vi "Spawn.vi"(9 "UID":string, 10 "Actor":refnum<class "Actor.lvclass">, 11 "Base Actor in":refnum<class "Base Actor.lvclass">) -> (0 "Error out":errorcluster, 3 "Base Actor out":refnum<class "Base Actor.lvclass">)   [LabVIEW 2025, in "jettl.lvlib" / "Actor.lvlib" / "Base Actor.lvclass"]
uses:
  Base Actor.lvclass
  Base Actor.lvclass/Base Actor.ctl
  Actor.vi
  Attributes/Attributes/Attributes.lvclass
  Spawn.ctl
  Actor.lvlib
  Actor/Actor.lvclass
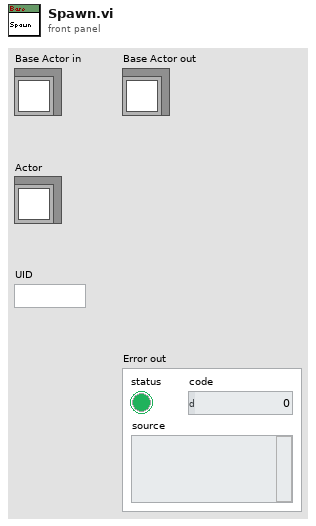
[diagram p1: front panel]
types:
  T1 = typedef "jettl.lvlib/Actor.lvlib/Spawn.ctl" = cluster{"UID":string, "Parent Attributes":refnum<class "Attributes.lvclass">, "Queue of Self Attributes":refnum<queue>, "Queue of Error":refnum<queue>}
  T2 = typedef "jettl.lvlib/Actor.lvlib/Base Actor.lvclass/Child Attributes Map.ctl" = map{string, refnum<class "Attributes.lvclass">}
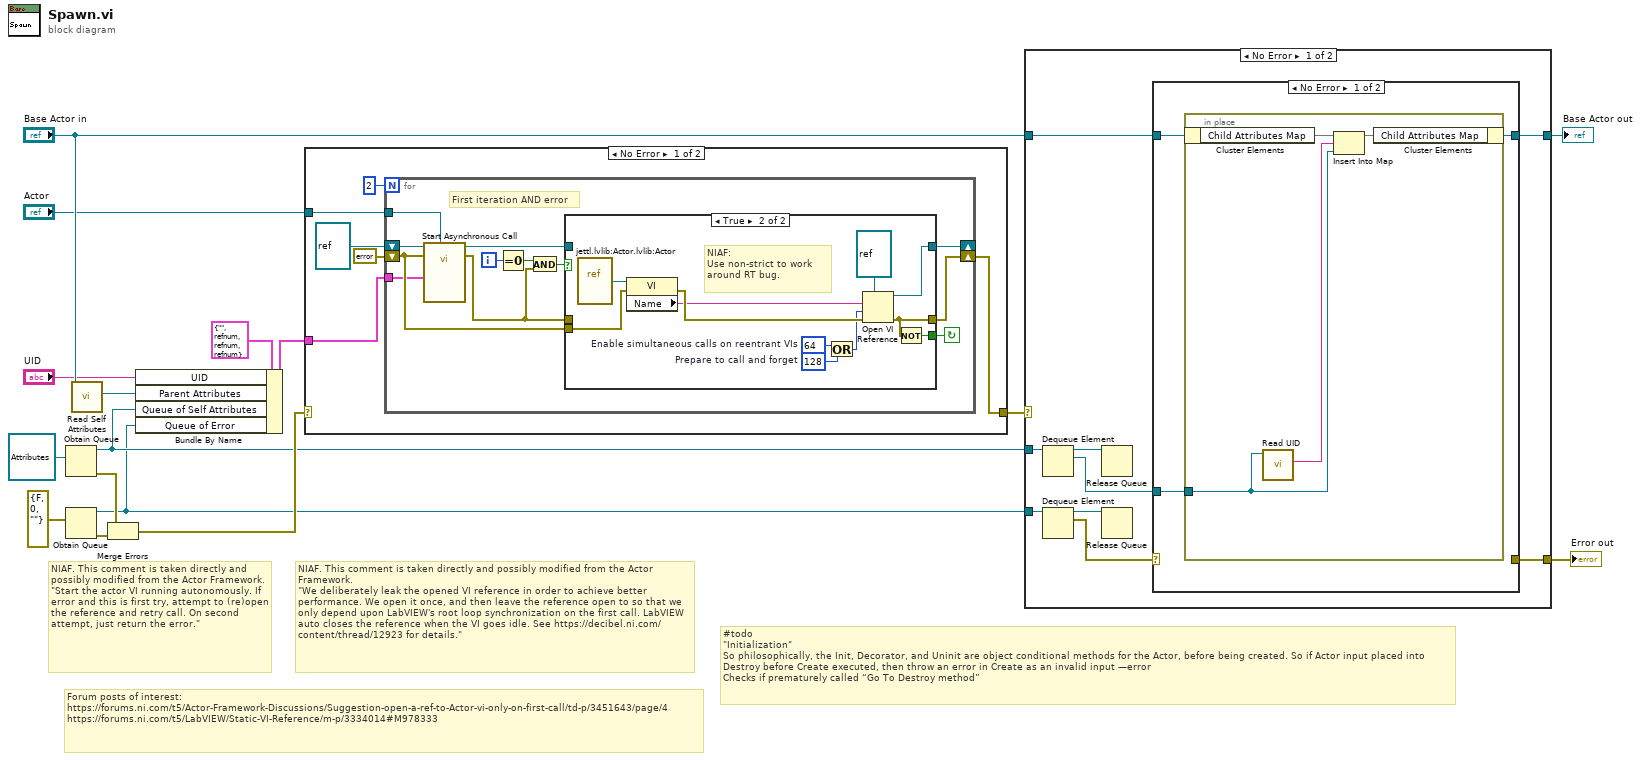
[diagram p0: block diagram]
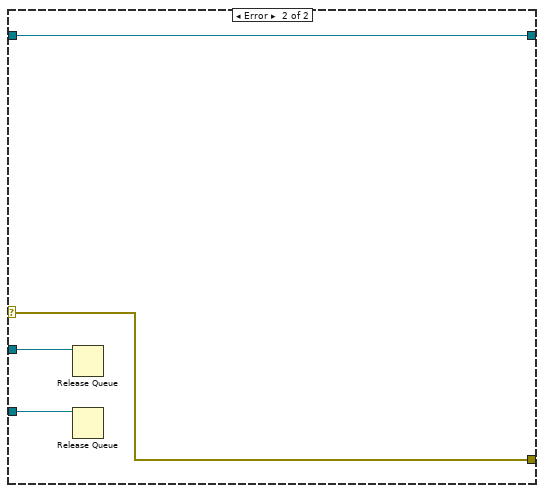
[diagram p3: hidden frame]
diagram:
  # "Forum posts of interest:\nhttps://forums.ni.com/t5/Actor-Framework-Discussions/Suggestion-open-a-ref-to-Actor-vi-only-on-first-call/td-p/3451643/page/4\nhttps://forums.ni.com/t5/LabVIEW/Static-VI-Reference/m-p/3334014#M978333"
  # "NIAF. This comment is taken directly and possibly modified from the Actor Framework.\n\"We deliberately leak the opened VI reference in order to achieve better performance. We open it once, and then leave the reference open to so that we only depend upon LabVIEW's root loop synchronization on the first call. LabVIEW auto closes the reference when the VI goes idle. See https://decibel.ni.com/content/thread/12923 for details.\""
  # "NIAF. This comment is taken directly and possibly modified from the Actor Framework.\n\"Start the actor VI running autonomously. If error and this is first try, attempt to (re)open the reference and retry call. On second attempt, just return the error.\""
  # "#todo\n\"Initialization\"\nSo philosophically, the Init, Decorator, and Uninit are object conditional methods for the Actor, before being created. So if Actor input placed into Destroy before Create executed, then throw an error in Create as an invalid input —error  \nChecks if prematurely called “Go To Destroy method”"
  n1 = Obtain Queue(element data type=refnum<class "Attributes.lvclass"> refnum ("jettl.lvlib:Attributes.lvlib:Attributes.lvclass")) -> (queue out=w2:refnum<queue>, error out=w9:errorcluster)  [unwired: 4 in, 1 out]
  n2 = Obtain Queue(element data type=errorcluster {"status"=FALSE, "code"=0, "source"=""} ("Error")) -> (queue out=w1:refnum<queue>, error out=w8:errorcluster)  [unwired: 4 in, 1 out]
  n3 = call-dynamic "Read Self Attributes.vi"("Base Actor in"="Base Actor in") -> ("Self Attributes"=w5:refnum<class "Attributes.lvclass">)  [unwired: 10 in]
  n4 = Merge Errors(w9, w8) -> (w10:errorcluster)
  n5 = Bundle By Name(cluster=T1 {"UID"="", "Parent Attributes"=refnum, "Queue of Self Attributes"=refnum, "Queue of Error"=refnum} ("Config Actor"), "UID"="UID", "Parent Attributes"=w5, "Queue of Self Attributes"=w2, "Queue of Error"=w1) -> (w3:T1)
  n6 = case shown="No Error" w10 {
    selector: w10 -> [_ w48]
    tunnel: [w17 w48] -> w13
    tunnel: "Actor" -> [w19 _]
    tunnel: w3 -> [w18 _]
    frame No Error {
      n7 = for {
        N: 2 -> [_]
        shift-right: [w34] -> _
        shift-left: refnum<vi> refnum -> [w33]
        shift-right: [w31] -> w17
        shift-left: errorcluster {"status"=FALSE, "code"=0, "source"=""} ("error out") -> [w27]
        tunnel: w19 -> [w24]
        tunnel: w18 -> [w23]
        i -> [w29]
        stop <- w28 continue-if-true
        # "First iteration AND error"
        n8 = call-by-ref "Start Asynchronous Call"(reference=w33, error in=w27, "Actor in"=w24, "Start"=w23) -> (reference out=w32:refnum<vi>, error out=w25:errorcluster)  [unwired: 8 in, 2 out]
        n9 = Equal To 0?(x=w29) -> (x = 0?=w26:bool)
        n10 = And(x=w26, y=w25) -> (x .and. y?=w30:bool)
        n11 = case shown="True" w30 {
          tunnel: [w36 w45] -> w34
          tunnel: [w35 w43] -> w31
          tunnel: w32 -> [w36 _]
          tunnel: w25 -> [w35 _]
          tunnel: [_ w44] -> w28
          tunnel: w27 -> [_ w42]
          frame False {
          }
          frame True {
            w37 = 64  # Enable simultaneous calls on reentrant VIs
            w39 = 128  # Prepare to call and forget
            # "NIAF:\nUse non-strict to work around RT bug."
            n12 = vi-ref "jettl.lvlib:Actor.lvlib:Actor.vi"() -> (w41:refnum<vi>)
            n13 = property class="VI"(reference=w41, error in=w42) -> (error out=w47:errorcluster, "Name"=w46:string)  [unwired: 1 out]
            n14 = Or(x=w37, y=w39) -> (x .or. y?=w38:i32)
            n15 = Open VI Reference(type specifier VI Refnum (for type only)=refnum<vi> refnum, vi path=w46, options=w38, error in (no error)=w47) -> (vi reference=w45:refnum<vi>, error out=w43:errorcluster)  [unwired: 2 in]
            n16 = Not(x=w43) -> (.not. x?=w44:bool)
          }
        }
      }
    }
    frame Error {
    }
  }
  n17 = case shown="No Error" w13 {
    selector: w13 -> [_ w67]
    tunnel: "Base Actor in" -> [w57 w69]
    tunnel: [w56 w69] -> w16
    tunnel: w2 -> [w55 w70]
    tunnel: w1 -> [w53 w68]
    tunnel: [w49 w67] -> w14
    frame No Error {
      n18 = Dequeue Element(queue=w55) -> (queue out=w54:refnum<queue>, element=w51:refnum<class "Attributes.lvclass">)  [unwired: 2 in, 2 out]
      n19 = Dequeue Element(queue=w53) -> (queue out=w52:refnum<queue>, element=w50:errorcluster)  [unwired: 2 in, 2 out]
      n20 = Release Queue(queue=w54) -> ()  [unwired: 2 in, 3 out]
      n21 = Release Queue(queue=w52) -> ()  [unwired: 2 in, 3 out]
      n22 = case shown="No Error" w50 {
        selector: w50 -> [_ w65]
        tunnel: w57 -> [w59 w66]
        tunnel: [w58 w66] -> w56
        tunnel: w51 -> [w60 _]
        tunnel: [_ w65] -> w49
        frame No Error {
          n23 = in-place {
            in-place-border: w60 -> [w61]
            n24 = in-place-cluster #1(w59) -> ("Child Attributes Map"=w64:T2)
            n25 = call-dynamic "Read UID.vi"("Attributes in"=w61) -> ("UID"=w62:string)  [unwired: 10 in]
            n26 = Insert Into Map(map in=w64, key=w62, value=w61) -> (map out=w63:T2)  [unwired: 2 out]
            n27 = in-place-cluster #1("Child Attributes Map"=w63) -> (w58:refnum<class "Base Actor.lvclass">)
          }
        }
        frame Error {
        }
      }
    }
    frame Error {
      n28 = Release Queue(queue=w70) -> ()  [unwired: 2 in, 3 out]
      n29 = Release Queue(queue=w68) -> ()  [unwired: 2 in, 3 out]
    }
  }
  "Base Actor out" <- w16
  "Error out" <- w14
